vi "Destroy Request Events.vi"(8 "error in":errorcluster) -> (0 "error out":errorcluster)   [LabVIEW 2026, in "Replay.lvlib"]
doc: "Destroy the requests user events, even if there is an incoming error.\n\n<b>NOTE</b>: The contents of this VI are automatically generated and modified by the <b>Tools > DQMH Consortium > DQMH</b> utilities. Consider using those utilities instead of making your own modifications to this VI.\n_____\nBased on DQMH Dev Tools: Project Template 7.1.2.1547."
uses:
  Replay.lvlib
panel:
  # "NOTE: The contents of this VI are automatically generated and modified by the Tools > DQMH Consortium > DQMH utilities. Consider using those utilities instead of making your own modifications to this VI."
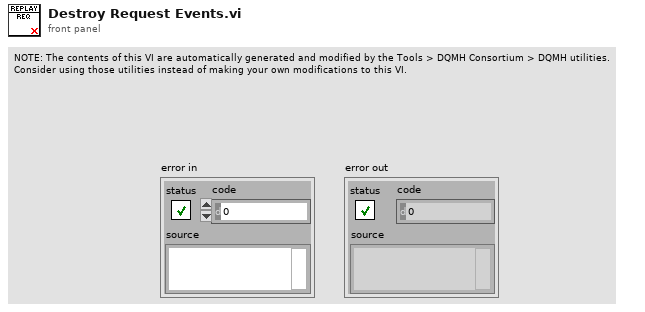
[diagram p1: front panel]
types:
  T1 = typedef "Replay.lvlib/Request Events--cluster.ctl" = cluster{"Stop Module":refnum<user-event>, "Show Panel":refnum<user-event>, "Hide Panel":refnum<user-event>, "Get Module Execution Status":refnum<user-event>, "Show Diagram":refnum<user-event>, "Set Run ID to Replay":refnum<user-event>}
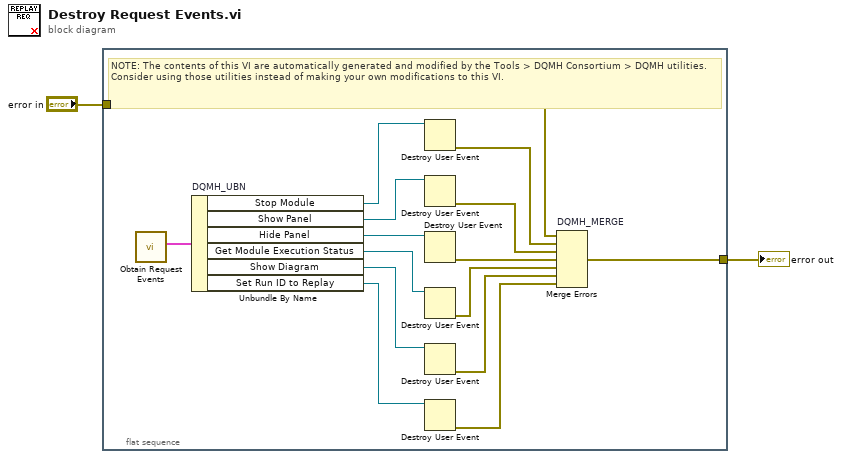
[diagram p0: block diagram]
diagram:
  n1 = flat-sequence {
    tunnel: [w16] -> w2
    tunnel: "error in" -> [w9]
    frame #0 {
      # "NOTE: The contents of this VI are automatically generated and modified by the Tools > DQMH Consortium > DQMH utilities. Consider using those utilities instead of making your own modifications to this VI."
      n2 = call "Obtain Request Events.vi"() -> ("Replay Request Events"=w15:T1)  [unwired: 10 in, 1 out]
      n3 = Unbundle By Name "DQMH_UBN"(w15) -> ("Stop Module"=w14:refnum<user-event>, "Show Panel"=w11:refnum<user-event>, "Hide Panel"=w10:refnum<user-event>, "Get Module Execution Status"=w7:refnum<user-event>, "Show Diagram"=w5:refnum<user-event>, "Set Run ID to Replay"=w3:refnum<user-event>)
      n4 = Destroy User Event(user event=w14) -> (error out=w17:errorcluster)  [unwired: 1 in]
      n5 = Destroy User Event(user event=w11) -> (error out=w13:errorcluster)  [unwired: 1 in]
      n6 = Destroy User Event(user event=w10) -> (error out=w12:errorcluster)  [unwired: 1 in]
      n7 = Destroy User Event(user event=w7) -> (error out=w8:errorcluster)  [unwired: 1 in]
      n8 = Destroy User Event(user event=w5) -> (error out=w6:errorcluster)  [unwired: 1 in]
      n9 = Destroy User Event(user event=w3) -> (error out=w4:errorcluster)  [unwired: 1 in]
      n10 = Merge Errors "DQMH_MERGE"(w9, w17, w13, w12, w8, w6, w4) -> (w16:errorcluster)
    }
  }
  "error out" <- w2
